vi "Get Default Output Stream List.vi"(8 "error in (no error)":errorcluster) -> (0 "error out":errorcluster, 3 "Output Streams":string[](array[string]))   [LabVIEW 2020, in "RandomNumberGenerator.lvlib" / "RandomNumberGenerator Controller.lvclass"]
doc: "<b>Get Default Output Stream List </b>\nThis method returns the output streams of this plugin. This information is used by PEF for linking up plugins based on the configuration."
uses:
  RandomNumberGenerator Controller.lvclass
  Read Output Streams.vi
  RandomNumberGenerator Controller.lvclass/RandomNumberGenerator Controller.ctl
panel:
  # "#via_ignore"
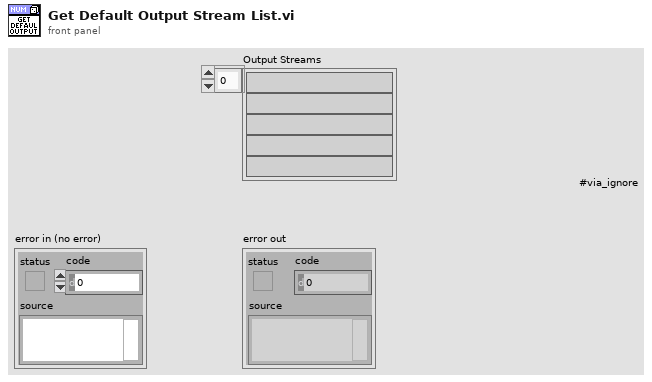
[diagram p1: front panel]
types:
  T1 = typedef "PluginSDK.lvlibp/Processing Element Specification.lvclass/Stream Specification.ctl" = cluster{"Name":string, "Channels":string[]}
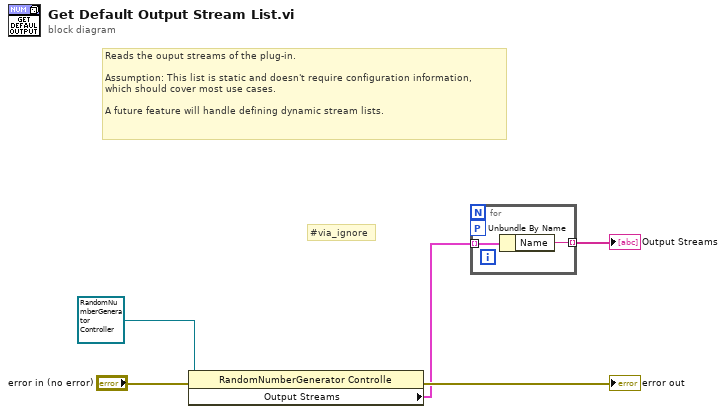
[diagram p0: block diagram]
diagram:
  # "#via_ignore"
  # "Reads the ouput streams of the plug-in.\n\nAssumption: This list is static and doesn't require configuration information,\nwhich should cover most use cases.\n\nA future feature will handle defining dynamic stream lists."
  n1 = property on="Property Node" class="RandomNumberGenerator Controlle"(reference=refnum<class "RandomNumberGenerator Controller.lvclass"> refnum ("ADAS PE Template Controller in"), error in="error in (no error)") -> (error out=→"error out":errorcluster, "Output Streams"=w1:T1[])  [unwired: 1 out]
  n2 = for {
    tunnel: w1 -> [w7] mode=indexing
    tunnel: [w6] -> w5 mode=indexing
    workers-P: _ -> [_]
    n3 = Unbundle By Name(w7) -> ("Name"=w6:string)
  }
  "Output Streams" <- w5
